vi "mission manager.vi"(0 "Spd Z1 In Cmd":i32, 1 "Msg 1 Z1 In":i32, 2 "Sonar Z1 In":i16, 5 "Alg In SF102 ck/in":i32, 7 "Msg 2 Z1 In":i32, 9 "Cros In SF102 ck/in":i32, 11 "Hdg Z1 In Cmd":i32, 12 "State Z1 In":i8) -> (3 "Msg 1 Z1 Out":i32, 4 "Spd Z1 Out Cmd 32.64 ck s/in cy":i32, 6 "Spd Out Cmd SF SF4.08 ck s/in cy":i32, 8 "Msg 2 Z1 Out":i32, 13 "Sonar Z1 Out":i16, 14 "State Z1 Out":i8, 15 "Hdg Z1 Out Cmd SF 5.33 ck/dg":i32)   [LabVIEW 2010, in "Test.lvrbt"]
uses:
  Test.lvrbt
  <vilib>/NXT/Block Support/NXT_InputPort.ctl
  <vilib>/NXT/Subs/MotorOutput.ctl
  <vilib>/NXT/Dual Mode Library/Sensors/Sonar_cm.vi
  <vilib>/NXT/Dual Mode Library/Motors/oldLightOn.vi
  <vilib>/NXT/Dual Mode Library/prims/maxAndMin/maxAndMin_int.vi
  GyroDrive/GyroDrive.lvrbt
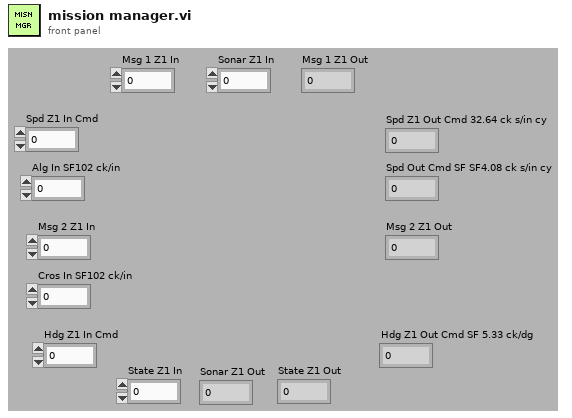
[diagram p1: front panel]
types:
  T1 = typedef "NXT_InputPort.ctl" = u8
  T2 = typedef "MotorOutput.ctl" = u8
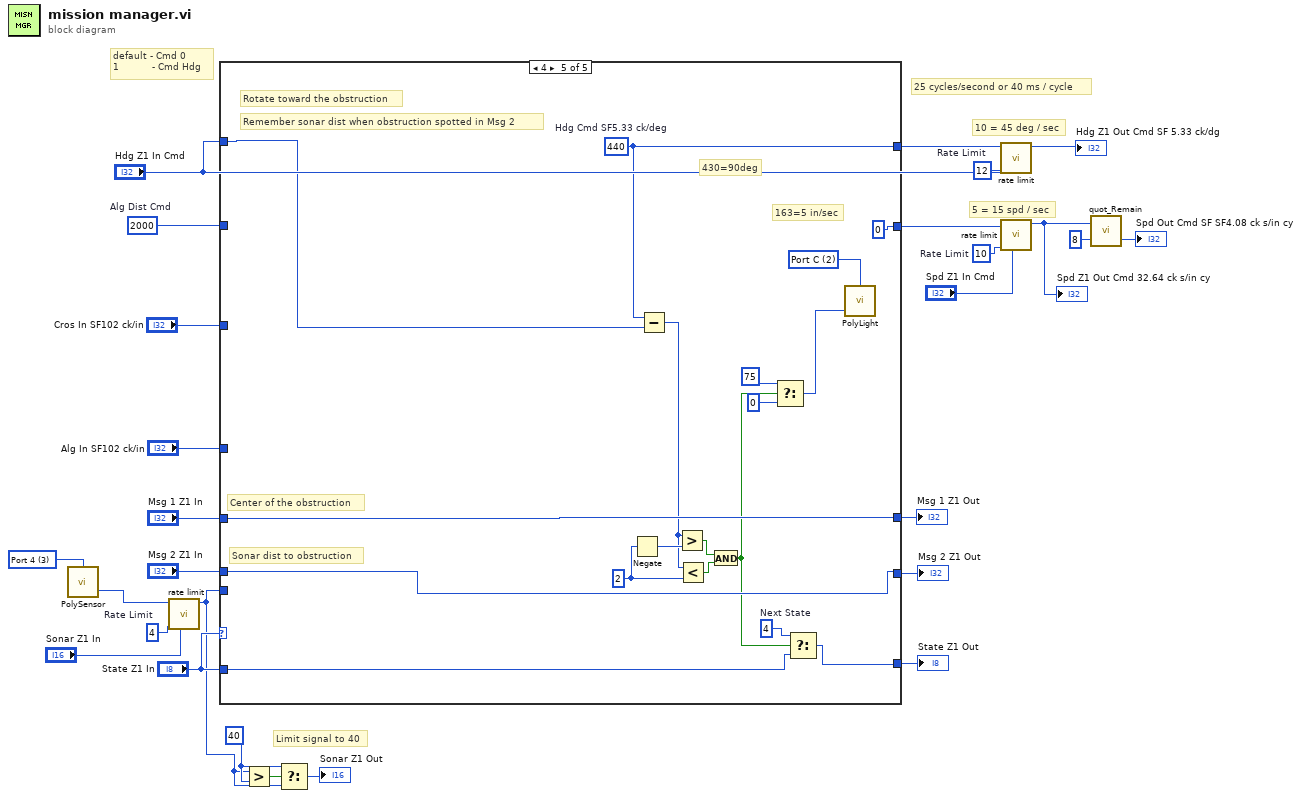
[diagram p0: block diagram]
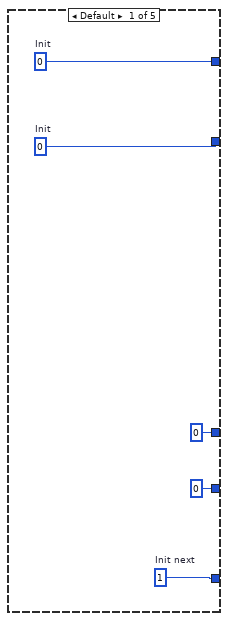
[diagram p2: hidden frame]
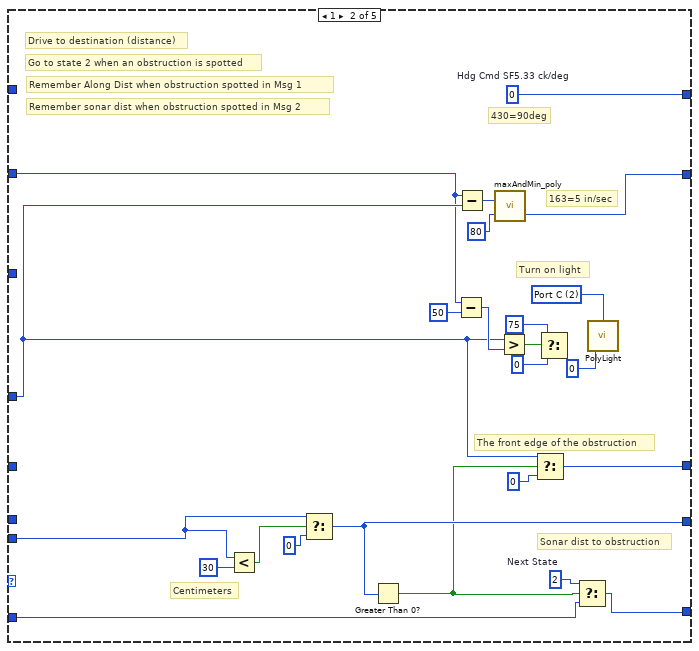
[diagram p3: hidden frame]
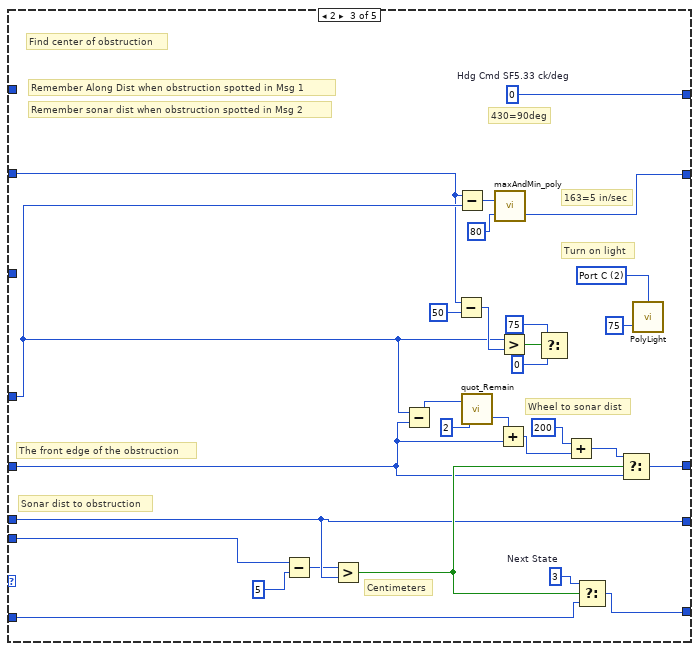
[diagram p4: hidden frame]
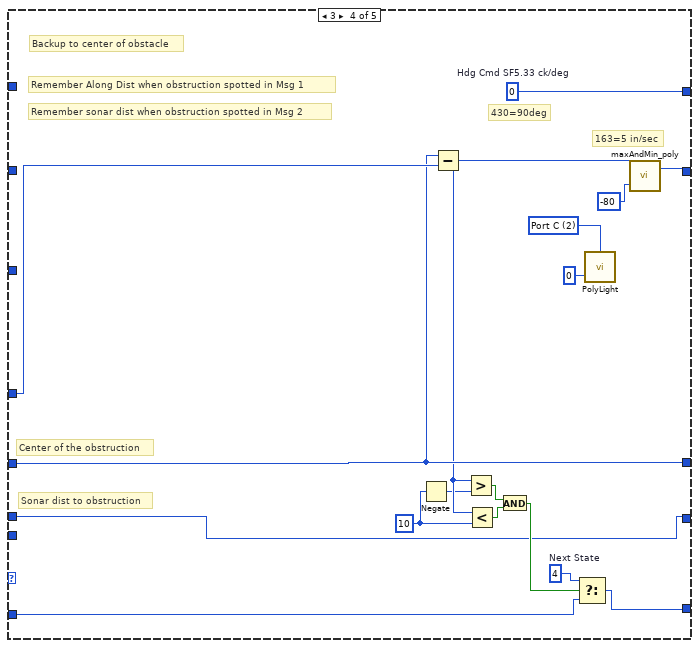
[diagram p5: hidden frame]
diagram:
  w3 = 40 ("y")
  w7 = 4  # Rate Limit
  w9 = T1 3 items=["Port 1", "Port 2", "Port 3", "Port 4"] ("Port (Port 4)")
  w10 = 2000  # Alg Dist Cmd
  w21 = 10  # Rate Limit
  w23 = 12  # Rate Limit
  # "Limit signal to 40"
  # "5 = 15 spd / sec"
  # "10 = 45 deg / sec"
  # "25 cycles/second or 40 ms / cycle"
  # "default - Cmd 0\n1           - Cmd Hdg"
  n1 = call-poly <vilib>:"PolySensor.vi"("Port (Port 4)"=w9) -> ("Distance (cm)"=w6:i16)  [unwired: 2 in, 1 out]
  n2 = call "rate limit.vi"("Z1 in"="Sonar Z1 In", "Rate Limit"=w7, "Signal In"=w6) -> ("Signal Z1 Out"=w1:i32)  [unwired: 8 in]
  n3 = case shown="4" "State Z1 In" {
    tunnel: "State Z1 In" -> [_ w36 w73 w98 w118]
    tunnel: [w31 w42 w78 w86 0 ("min(x,y)")] -> w24
    tunnel: [w32 w56 w85 w102 w109] -> w25
    tunnel: "Cros In SF102 ck/in" -> [_ _ _ _ _]
    tunnel: "Alg In SF102 ck/in" -> [_ w38 w72 w97 _]
    tunnel: "Hdg Z1 In Cmd" -> [_ _ _ _ w108]
    tunnel: [0 ("Msg 1 Z1 In") w40 w70 w96 w117] -> w15
    tunnel: "Msg 1 Z1 In" -> [_ _ w66 w96 w117]
    tunnel: [w28 w43 w74 w99 w119] -> w13
    tunnel: [0 ("Msg 2 Z1 In") w41 w63 w89 w112] -> w12
    tunnel: "Msg 2 Z1 In" -> [_ _ w63 w89 w112]
    tunnel: w10 -> [_ w35 w64 _ _]
    tunnel: w1 -> [_ w33 w61 _ _]
    frame Default {
      w28 = 1  # Init next
      w31 = 0  # Init
      w32 = 0  # Init
    }
    frame 1 {
      w44 = i8 2  # Next State
      w53 = T2 2 items=["Port A"=0, "Port B"=1, "Port C"=2, "Ports A & B"=4, "Ports A & C"=5, "Ports B & C"=6, "All Ports"=3] ("Output Port (All Ports)")
      w56 = 0  # Hdg Cmd SF5.33 ck/deg
      # "Sonar dist to obstruction"
      # "The front edge of the obstruction"
      # "Remember sonar dist when obstruction spotted in Msg 2"
      # "Remember Along Dist when obstruction spotted in Msg 1"
      # "Go to state 2 when an obstruction is spotted"
      # "Centimeters"
      # "Drive to destination (distance)"
      # "163=5 in/sec"
      # "Turn on light"
      # "430=90deg"
      n4 = Less?(x=w33, y=i16 30) -> (x < y?=w46:bool)
      n5 = Select(t=w33, s=w46, f=i16 0) -> (s? t:f=w41:i32)
      n6 = Greater Than 0?(x=w41) -> (x > 0?=w39:bool)
      n7 = Subtract(x=w35, y=50) -> (x-y=w48:i32)
      n8 = Subtract(x=w35, y=w38) -> (x-y=w50:i32)
      n9 = call-poly <vilib>:"maxAndMin_poly.vi"("y"=80, "x"=w50) -> ("min(x,y)"=w42:i32)  [unwired: 1 out]
      n10 = Greater?(x=w38, y=w48) -> (0:w55:bool)
      n11 = Select(t=w38, s=w39, f=0) -> (s? t:f=w40:i32)
      n12 = Select(t=75, s=w55, f=0) -> ()  [unwired: 1 out]
      n13 = Select(t=w44, s=w39, f=w36) -> (s? t:f=w43:i8)
      n14 = call-poly <vilib>:"PolyLight.vi"("Power (75)"=0, "Output Port (All Ports)"=w53) -> ()  [unwired: 2 in, 1 out]
    }
    frame 2 {
      w75 = i8 3  # Next State
      w82 = T2 2 items=["Port A"=0, "Port B"=1, "Port C"=2, "Ports A & B"=4, "Ports A & C"=5, "Ports B & C"=6, "All Ports"=3] ("Output Port (All Ports)")
      w85 = 0  # Hdg Cmd SF5.33 ck/deg
      # "Wheel to sonar dist"
      # "Sonar dist to obstruction"
      # "The front edge of the obstruction"
      # "Remember sonar dist when obstruction spotted in Msg 2"
      # "Remember Along Dist when obstruction spotted in Msg 1"
      # "Centimeters"
      # "Find center of obstruction"
      # "163=5 in/sec"
      # "Turn on light"
      # "430=90deg"
      n15 = Subtract(x=w61, y=i16 5 ("x")) -> (x-y=w62:i32)
      n16 = Greater?(x=w62, y=w63) -> (0:w71:bool)
      n17 = Subtract(x=w72, y=w66) -> (x-y=w68:i32)
      n18 = Subtract(x=w64, y=50) -> (x-y=w76:i32)
      n19 = Subtract(x=w64, y=w72) -> (x-y=w79:i32)
      n20 = call <vilib>:"quot_Remain.vi"("y"=2, "x"=w68) -> ("floor(x/y)"=w67:i32)  [unwired: 1 out]
      n21 = call-poly <vilib>:"maxAndMin_poly.vi"("y"=80, "x"=w79) -> ("min(x,y)"=w78:i32)  [unwired: 1 out]
      n22 = Add(x=w67, y=w66) -> (x+y=w58:i32)
      n23 = Greater?(x=w72, y=w76) -> (0:w84:bool)
      n24 = Select(t=75, s=w84, f=0) -> ()  [unwired: 1 out]
      n25 = Add(x=200, y=w58) -> (x+y=w59:i32)
      n26 = Select(t=w75, s=w71, f=w73) -> (s? t:f=w74:i8)
      n27 = Select(t=w59, s=w71, f=w66) -> (s? t:f=w70:i32)
      n28 = call-poly <vilib>:"PolyLight.vi"("Power (75)"=75, "Output Port (All Ports)"=w82) -> ()  [unwired: 2 in, 1 out]
    }
    frame 3 {
      w88 = T2 2 items=["Port A"=0, "Port B"=1, "Port C"=2, "Ports A & B"=4, "Ports A & C"=5, "Ports B & C"=6, "All Ports"=3] ("Output Port (All Ports)")
      w94 = 10 ("y")
      w100 = i8 4  # Next State
      w102 = 0  # Hdg Cmd SF5.33 ck/deg
      # "Remember sonar dist when obstruction spotted in Msg 2"
      # "Backup to center of obstacle"
      # "Sonar dist to obstruction"
      # "Center of the obstruction"
      # "Remember Along Dist when obstruction spotted in Msg 1"
      # "163=5 in/sec"
      # "430=90deg"
      n29 = Negate(x=w94) -> (-x=w93:i32)
      n30 = Subtract(x=w96, y=w97) -> (x-y=w95:i32)
      n31 = Greater?(x=w95, y=w93) -> (0:w91:bool)
      n32 = Less?(x=w95, y=w94) -> (x < y?=w92:bool)
      n33 = And(x=w91, y=w92) -> (x .and. y?=w90:bool)
      n34 = Select(t=w100, s=w90, f=w98) -> (s? t:f=w99:i8)
      n35 = call-poly <vilib>:"PolyLight.vi"("Power (75)"=0, "Output Port (All Ports)"=w88) -> ()  [unwired: 2 in, 1 out]
      n36 = call-poly <vilib>:"maxAndMin_poly.vi"("y"=-80, "x"=w95) -> ("max(x,y)"=w86:i32)  [unwired: 1 out]
    }
    frame 4 {
      w111 = T2 2 items=["Port A"=0, "Port B"=1, "Port C"=2, "Ports A & B"=4, "Ports A & C"=5, "Ports B & C"=6, "All Ports"=3] ("Output Port (All Ports)")
      w116 = 2 ("y")
      w120 = i8 4  # Next State
      w109 = 440  # Hdg Cmd SF5.33 ck/deg
      # "Remember sonar dist when obstruction spotted in Msg 2"
      # "Rotate toward the obstruction"
      # "Sonar dist to obstruction"
      # "Center of the obstruction"
      # "163=5 in/sec"
      # "430=90deg"
      n37 = Negate(x=w116) -> (-x=w115:i32)
      n38 = Subtract(x=w109, y=w108) -> (x-y=w107:i32)
      n39 = Greater?(x=w107, y=w115) -> (0:w113:bool)
      n40 = Less?(x=w107, y=w116) -> (x < y?=w114:bool)
      n41 = And(x=w113, y=w114) -> (x .and. y?=w104:bool)
      n42 = Select(t=i8 75 ("Next State"), s=w104, f=i8 0) -> (s? t:f=w103:i8)
      n43 = Select(t=w120, s=w104, f=w118) -> (s? t:f=w119:i8)
      n44 = call-poly <vilib>:"PolyLight.vi"("Power (75)"=w103, "Output Port (All Ports)"=w111) -> ()  [unwired: 2 in, 1 out]
    }
  }
  "State Z1 Out" <- w13
  "Msg 1 Z1 Out" <- w15
  "Msg 2 Z1 Out" <- w12
  n45 = Greater?(x=w1, y=w3) -> (0:w4:bool)
  n46 = Select(t=w3, s=w4, f=w1) -> (s? t:f=→"Sonar Z1 Out":i32)
  n47 = call "rate limit.vi"("Z1 in"="Hdg Z1 In Cmd", "Rate Limit"=w23, "Signal In"=w25) -> ("Signal Z1 Out"=→"Hdg Z1 Out Cmd SF 5.33 ck/dg":i32)  [unwired: 8 in]
  n48 = call "rate limit.vi"("Z1 in"="Spd Z1 In Cmd", "Rate Limit"=w21, "Signal In"=w24) -> ("Signal Z1 Out"=w18:i32)  [unwired: 8 in]
  "Spd Z1 Out Cmd 32.64 ck s/in cy" <- w18
  n49 = call <vilib>:"quot_Remain.vi"("y"=8, "x"=w18) -> ("floor(x/y)"=→"Spd Out Cmd SF SF4.08 ck s/in cy":i32)  [unwired: 1 out]
